vi "SICK Only Diagnostic.vi"() -> ()   [LabVIEW 2009]
uses:
  <vilib>/userDefined/High Color/nirio_resource_hc.ctl
  <vilib>/rvi/interface/nirviOpenFPGA/nirviOpenFPGA.xnode
  FPGA Bitfiles/Q_IGVC_2010.lvproj_FPGA Target_SICK Only.vi.lvbitx
  <vilib>/FPGAPlugInAG/cRIO-9113/nirviIntfOpen_cRIO-9113.vi
  <vilib>/Platform/TimedLoop/XDataNode/XDataNode.xnode
  <vilib>/Platform/TimedLoop/XDataNode/loadlvalarms.vi
  <vilib>/Platform/TimedLoop/XDataNode/timing_clust.ctl
  <vilib>/Platform/TimedLoop/XDataNode/nitl_modes.ctl
  <vilib>/Platform/TimedLoop/XDataNode/wakeup.ctl
  <vilib>/rvi/interface/nirviReadWriteControl/nirviReadWriteControl.xnode
  <vilib>/Utility/error.llb/Error Cluster From Error Code.vi
  <vilib>/rvi/errors/niLvFpgaAdjustHostInterfaceError.vi
  <vilib>/rvi/interface/common/niFpgaNodeNameForErrorReporting.ctl
  <vilib>/rvi/errors/niLvFpgaWhatHappensToTopLevelVI.ctl
  <vilib>/Platform/TimedLoop/XDataNode/XDNodeRunTimeDep.lvlib
  SICK Only FPGA Ref.ctl
  NiRioSrv.dll
panel:
  out "Initialization success":bool
  out "Loop Period":u32
  in  "stop":bool
  out "Waveform Graph":u16[](graph)
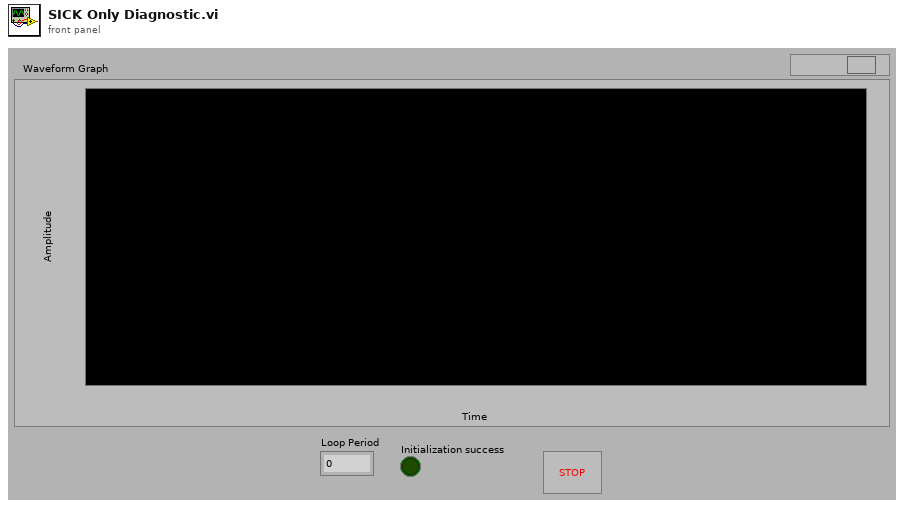
[diagram p1: front panel]
types:
  T1 = typedef "nirio_resource_hc.ctl" = tag
  T2 = typedef "SICK Only FPGA Ref.ctl" = refnum<k20>
  T3 = typedef "XDNodeRunTimeDep.lvlib/timing_clust.ctl" = cluster{"Expected End [f-1]":u64, "Actual End [f-1]":u64, "Finished Late? [f-1]":bool, "Expected End [i-1]":u64, "Actual End [i-1]":u64, "Finished Late? [i-1]":bool, "Expected Start [i]":u64, "Actual Start [i]":u64, "Expected Start [f]":u64, "Actual Start [f]":u64, "Source Name":string, "Structure Name":string, "Period":i64, "Deadline":i64, "Offset":i64, "Start":i64, "Priority":i32, "Timeout":i32, "Mode":T4, "Wakeup Reason":T5, "Error":errorcluster, "Source Type":string, "Secondary Source Type":string, "Global End Time":u64, "Global Start Time":u64, "Frame Duration":u64, "Iteration Duration":u64, "Assigned CPU":i32, "I/O Scan Engine Mode":u32}
  T4 = typedef "XDNodeRunTimeDep.lvlib/nitl_modes.ctl" = enum32{"No Change", "Process missed periods, maintain original phase", "Discard missed periods, maintain original phase", "Process missed periods, ignore original phase", "Discard missed periods, ignore original phase"}
  T5 = typedef "XDNodeRunTimeDep.lvlib/wakeup.ctl" = enum32{"Normal", "Aborted", "Asynchronous wakeup", "Timing source error", "Timed loop error", "Timeout"}
  T6 = typedef "niFpgaNodeNameForErrorReporting.ctl" = enum16{"Open FPGA VI Reference", "Read/Write Control", "Invoke Method: Abort", "Invoke Method: Acknowledge IRQ", "Invoke Method: Download", "Invoke Method: FIFO.Configure", "Invoke Method: FIFO.Read", "Invoke Method: FIFO.Start", "Invoke Method: FIFO.Stop", "Invoke Method: FIFO.Write", "Invoke Method: Reset", "Invoke Method: Run", "Invoke Method: Wait on IRQ", "Close FPGA VI Reference"}
  T7 = typedef "niLvFpgaWhatHappensToTopLevelVI.ctl" = enum16{"top level VI scripted behind XNode", "top level VI inlined behind XNode"}
  T8 = typedef "SICK Array.ctl" = u16[]
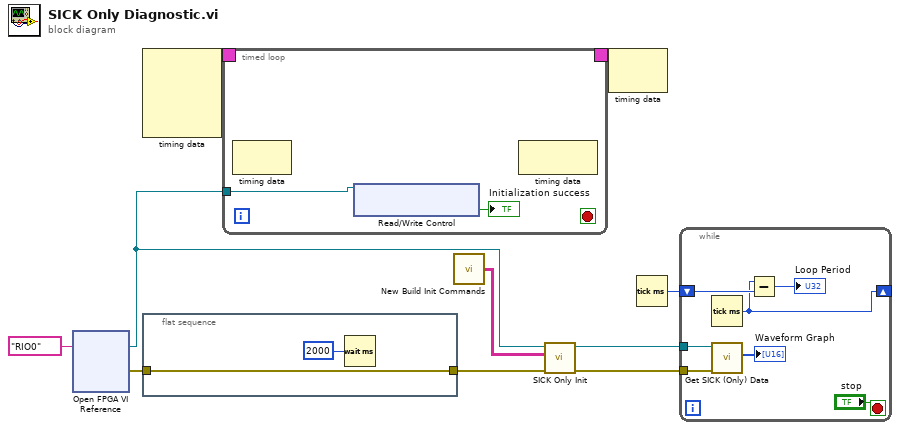
[diagram p0: block diagram]
diagram:
  n1 = xnode "Open FPGA VI Reference"("resource name"=T1 "RIO0") -> ("FPGA VI Reference Out"=w1:T2, "error out"=w4:errorcluster)  [unwired: 1 in]
  n2 = node-c288() -> (w7:T3)  [unwired: 4 in]
  n3 = flat-sequence {
    tunnel: [w12] -> w5
    tunnel: w4 -> [w12]
    frame #0 {
      n4 = Wait (ms)(milliseconds to wait=u32 2000) -> ()  [unwired: 1 out]
    }
  }
  n5 = timed-loop {
    timing: w7 -> [_]
    timing-out: [_] -> w6
    tunnel: w1 -> [w14]
    stop <- _ stop-if-true
    n6 = node-c288() -> ()  [unwired: 1 in, 1 out]
    n7 = xnode "Read/Write Control"("FPGA VI Reference In"=w14) -> ("Initialization success"=→"Initialization success":bool)  [unwired: 1 in, 2 out]
    n8 = node-c288() -> ()  [unwired: 1 in, 1 out]
  }
  n9 = call "New Build Init Commands.vi"() -> ("SICK Commands"=w2:string[][])
  n10 = call "SICK Only Init.vi"("error in"=w5, "SICK Commands"=w2, "SICK Only ref in"=w1) -> ("error out"=w8:errorcluster, "SICK Only ref out"=w9:T2)  [unwired: 6 in, 1 out]
  n11 = node-c288(w6) -> ()  [unwired: 1 out]
  n12 = Tick Count (ms)() -> (millisecond timer value=w3:u32)
  n13 = while {
    tunnel: w9 -> [w64]
    tunnel: w8 -> [w63]
    shift-right: [w59] -> _
    shift-left: w3 -> [w60]
    stop <- "stop" stop-if-true
    n14 = Tick Count (ms)() -> (millisecond timer value=w59:u32)
    n15 = call "Get SICK (Only) Data.vi"("error in"=w63, "SICK Only ref in"=w64) -> ("SICK Data"=→"Waveform Graph":T8)  [unwired: 7 in, 2 out]
    n16 = Subtract(x=w59, y=w60) -> (x-y=→"Loop Period":u32)
  }
